vi "RT_Control_Adrian_ESP_NoTrigger.vi"(10 "rt fifo":refnum<k33>, 11 "Parameters":T1={"N_chan"=0, "Input Rate (Hz)"=0.0, "Acq Time (s)"=0.0, "NumOfWarmupIters"=0, "Size fifo"=0, "Period NCL (ms)"=0, "Timeout fifo Read"=0, "Size Sent Array"=0, "Output offsets"=[], "Input offsets"=[0.0, 0.0, 0.0, 0.0, 0.0, 0.0, 0.0, 0.0]}) -> (0 "error out":errorcluster, 2 "Delayed Cycles":dbl)   [LabVIEW 2021]
uses:
  ClosedLoopFlapV3/parametersRT.ctl
  <vilib>/DAQmx/write.llb/DAQmx Write (Analog 1D DBL NChan 1Samp).vi
  <vilib>/DAQmx/read.llb/DAQmx Read (Analog 1D DBL NChan 1Samp).vi
  <vilib>/DAQmx/configure/timing.llb/DAQmx Timing (Sample Clock).vi
  <vilib>/DAQmx/miscellaneous.llb/DAQmx Fill In Error Info.vi
  <resource>/objmgr/daqmx.rc
panel:
  out "timed out?":bool
  out "# elements":u32
  out "data":dbl[](array[numeric]) format="%0.2f"
  out "Numeric":i32
  out "output array":dbl[](array[numeric])
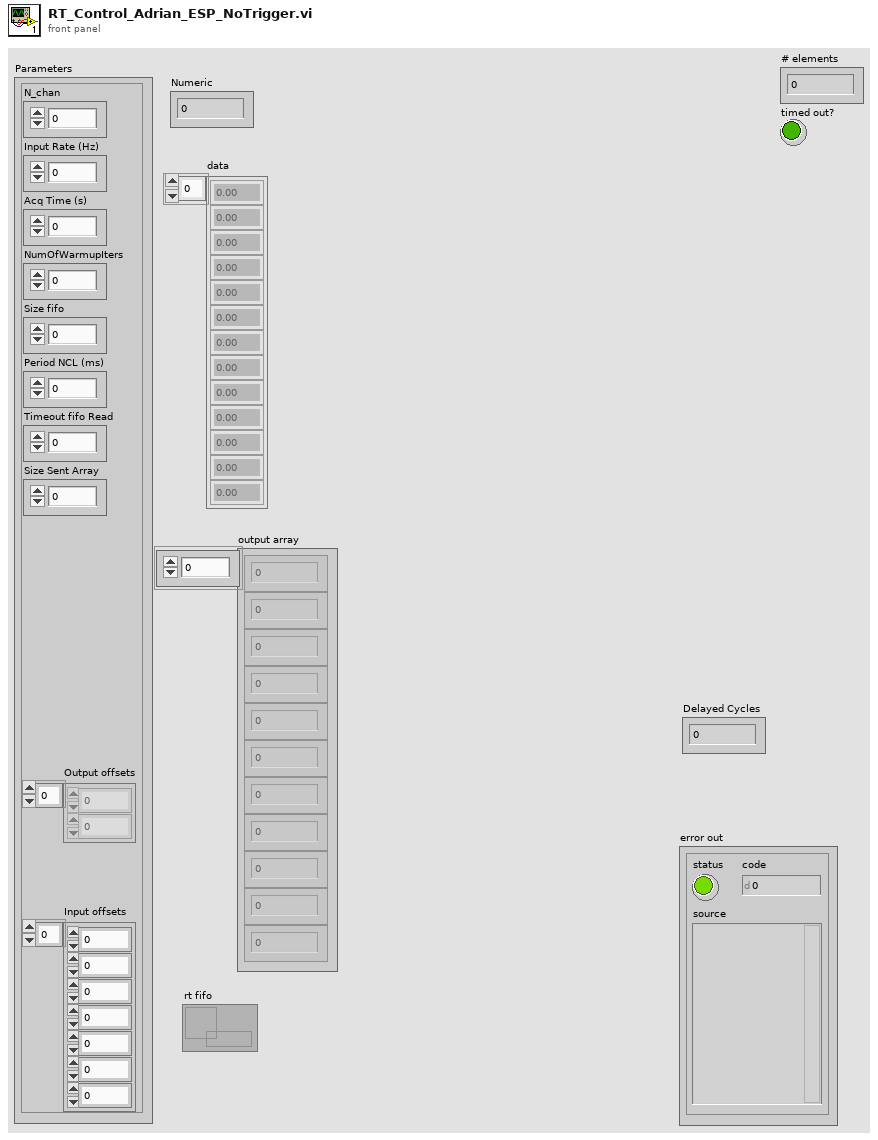
[diagram p1: front panel]
types:
  T1 = typedef "parametersRT.ctl" = cluster{"N_chan":u32, "Input Rate (Hz)":dbl, "Acq Time (s)":dbl, "NumOfWarmupIters":u32, "Size fifo":u32, "Period NCL (ms)":i64, "Timeout fifo Read":i32, "Size Sent Array":i32, "Output offsets":dbl[], "Input offsets":dbl[]}
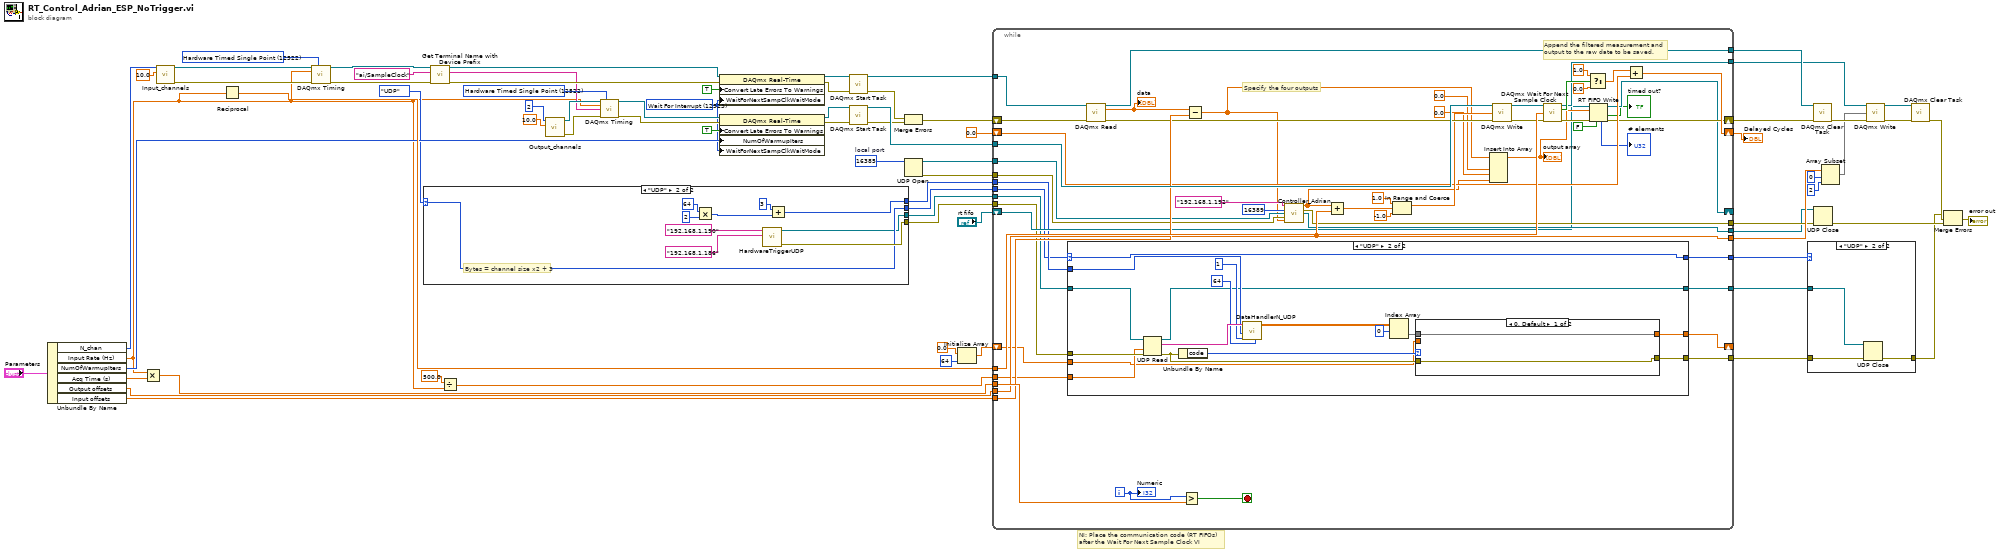
[diagram p0: block diagram]
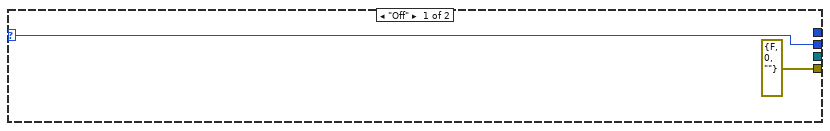
[diagram p3: hidden frame]
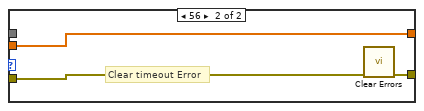
[diagram p5: hidden frame]
diagram:
  w31 = u16 16385  # local port
  w38 = 12522 items=["Finite Samples"=10178, "Continuous Samples"=10123, "Hardware Timed Single Point"=12522] ("sample mode")
  w46 = 12523 items=["Wait For Interrupt"=12523, "Poll"=12524, "Yield"=12525] ("WaitForNextSampClkWaitMode")
  w72 = 12522 items=["Finite Samples"=10178, "Continuous Samples"=10123, "Hardware Timed Single Point"=12522] ("sample mode")
  # "NI: Place the communication code (RT FIFOs) \nafter the Wait For Next Sample Clock VI"
  n1 = Unbundle By Name("Parameters") -> ("N_chan"=w57:u32, "Input Rate (Hz)"=w6:dbl, "NumOfWarmupIters"=w58:u32, "Acq Time (s)"=w65:dbl, "Output offsets"=w56:dbl[], "Input offsets"=w47:dbl[])
  n2 = Multiply(x=w6, y=w65) -> (x*y=w25:dbl)
  n3 = call "Input_channels.vi"("Range"=10.0, "nchan"=w57) -> ("error out"=w40:errorcluster, "Refnum out"=w39:refnum<k21>)  [unwired: 8 in]
  n4 = Reciprocal(x=w6) -> (1/x=w71:dbl)
  n5 = call-poly <vilib>:"DAQmx Timing.vi"("task/channels in"=w39, "sample mode"=w38, "rate"=w6, "error in"=w40) -> ("task out"=w19:refnum<k21>, "error out"=w21:errorcluster)  [unwired: 10 in]
  n6 = case shown="\"UDP\"" enum16{"Off", "UDP"}."UDP" {
    selector: enum16{"Off", "UDP"}."UDP" -> [w75 w78]
    tunnel: [_ w81] -> w12
    tunnel: [errorcluster {"status"=FALSE, "code"=0, "source"=""} ("error constant") w79] -> w14
    tunnel: [w75 w78] -> w11
    tunnel: [_ w77] -> w13
    frame "Off" {
    }
    frame "UDP" {
      # "Bytes = channel size x2 + 3"
      n7 = Multiply(x=64, y=2) -> (x*y=w84:i32)
      n8 = call "HardwareTriggerUDP.vi"("Local IP address"="192.168.1.186" ("Hardware Trigger"), "Remote IP address"="192.168.1.190" ("IP address")) -> ("error out"=w79:errorcluster, "connection ID out"=w77:refnum<k16>)  [unwired: 8 in]
      n9 = Add(x=3, y=w84) -> (x+y=w81:i32)
    }
  }
  n10 = call "Get Terminal Name with Device Prefix.vi"("error in (no error)"=w21, "Local Terminal Name"="ai/SampleClock", "task/channels in"=w19) -> ("error out"=w20:errorcluster, "Terminal Name with Device Prefix"=w17:tag, "task out"=w18:refnum<k21>)  [unwired: 6 in]
  n11 = Divide(x=500.0, y=w6) -> (x/y=w5:dbl)
  n12 = call "Output_channels.vi"("Range"=10.0 ("Maximum Value"), "nchan"=2) -> ("error out"=w62:errorcluster, "Refnum out"=w61:refnum<k21>)  [unwired: 8 in]
  n13 = call-poly <vilib>:"DAQmx Timing.vi"("task/channels in"=w61, "sample mode"=w72, "rate"=w6, "source"=w17, "error in"=w62) -> ("task out"=w70:refnum<k21>, "error out"=w69:errorcluster)  [unwired: 9 in]
  n14 = property class="DAQmx Real-Time"(reference=w18, error in=w20, "Convert Late Errors To Warnings"=TRUE, "WaitForNextSampClkWaitMode"=w46) -> (reference out=w35:refnum<k21>, error out=w34:errorcluster)
  n15 = property class="DAQmx Real-Time"(reference=w70, error in=w69, "Convert Late Errors To Warnings"=TRUE, "NumOfWarmupIters"=w58, "WaitForNextSampClkWaitMode"=w46) -> (reference out=w66:refnum<k21>, error out=w43:errorcluster)
  n16 = call <vilib>:"DAQmx Start Task.vi"("task/channels in"=w35, "error in"=w34) -> ("task out"=w64:refnum<k21>, "error out"=w33:errorcluster)  [unwired: 12 in]
  n17 = call <vilib>:"DAQmx Start Task.vi"("task/channels in"=w66, "error in"=w43) -> ("task out"=w63:refnum<k21>, "error out"=w42:errorcluster)  [unwired: 12 in]
  n18 = Merge Errors(w33, w42) -> (w32:errorcluster)
  n19 = UDP Open(11:w31) -> (port=w29:refnum<k16>, 0:w30:errorcluster)  [unwired: 4 in, 1 out]
  n20 = Initialize Array(0.0, 64) -> (w8:dbl[])
  n21 = while {
    shift-right: [w105] -> w41
    shift-left: w32 -> [w123]
    shift-right: [w135] -> w73
    shift-left: 0.0 ("f") -> [w110]
    tunnel: w71 -> [w133]
    tunnel: w25 -> [w131]
    tunnel: w63 -> [w129]
    tunnel: [w124] -> w67
    tunnel: w64 -> [w125]
    tunnel: [w127] -> w55
    tunnel: w56 -> [w118]
    tunnel: [w118] -> w50
    tunnel: w47 -> [w126]
    tunnel: w30 -> [w116]
    tunnel: w29 -> [w115]
    tunnel: [w114] -> w28
    tunnel: [w113] -> w27
    shift-right: [w101] -> _
    shift-left: "rt fifo" -> [w102]
    tunnel: w14 -> [w95]
    tunnel: w13 -> [w94]
    tunnel: w12 -> [w93]
    tunnel: w11 -> [w92]
    tunnel: w5 -> [w90]
    tunnel: [w89] -> w4
    tunnel: [w88] -> w3
    tunnel: [w87] -> w2
    shift-right: [w86] -> _
    shift-left: w8 -> [w91]
    i -> [w108]
    stop <- w132 stop-if-true
    # "Append the filtered measurement and \noutput to the raw date to be saved."
    # "Specify the four outputs"
    n22 = case shown="\"UDP\"" w92 {
      selector: w92 -> [w142 w156]
      tunnel: w93 -> [_ w158]
      tunnel: w95 -> [w141 w157]
      tunnel: [w141 w150] -> w88
      tunnel: [w142 w156] -> w87
      tunnel: [w139 w146] -> w86
      tunnel: w90 -> [_ w147]
      tunnel: w94 -> [w140 w149]
      tunnel: [w140 w148] -> w89
      tunnel: w91 -> [w139 w145]
      frame "Off", Default {
      }
      frame "UDP" {
        n23 = UDP Read(connection ID=w149, timeout ms (25000)=w147, 8:w157) -> (data out=w159:string, error out=w151:errorcluster, 3:w148:refnum<k16>)  [unwired: 1 in, 2 out]
        n24 = Unbundle By Name(w151) -> ("code"=w152:i32)
        n25 = call "DataHandlerN_UDP.vi"("Data Cycles Per Buffer"=1, "Rx Packet Byte size"=w158, "data out"=w159, "Nchan"=64) -> ("Data"=w143:sgl[][])  [unwired: 1 in, 4 out]
        n26 = Index Array(array=w143, index (row)=0 ("Data Cycles Per Buffer")) -> (element=w144:sgl[])  [unwired: 1 in]
        n27 = case shown="0, Default" w152 {
          tunnel: w151 -> [w161 w164]
          tunnel: [w161 w163] -> w150
          tunnel: w144 -> [w160 _]
          tunnel: [w160 w162] -> w146
          tunnel: w145 -> [_ w162]
          frame 0, Default {
          }
          frame 56 {
            # "Clear timeout Error"
            n28 = call <vilib>:"Clear Errors.vi"("error in (no error)"=w164) -> ("error out"=w163:errorcluster)  [unwired: 5 in, 1 out]
          }
        }
      }
    }
    n29 = call-poly <vilib>:"DAQmx Read.vi"("task/channels in"=w125, "error in"=w123) -> ("task out"=w124:refnum<k21>, "data"=w107:dbl[], "error out"=w122:errorcluster)  [unwired: 11 in]
    "data" <- w107
    n30 = Greater?(x=w108, y=w131) -> (0:w132:bool)
    n31 = Subtract(x=w107, y=w126) -> (x-y=w109:dbl[])
    n32 = call "Controller_Adrian.vi"("name 2"="192.168.1.192", "port or service name"=u16 16389, "connection ID"=w115, "error in (no error)"=w116, "x"=w109) -> ("*(type *) &x"=w100:dbl[], "error out"=w114:errorcluster, "connection ID out"=w113:refnum<k16>)  [unwired: 8 in]
    n33 = Add(x=w100, y=w118) -> (x+y=w120:dbl[])
    n34 = In Range and Coerce(upper limit=1.0, x=w120, lower limit=-1.0) -> (coerced(x)=w117:dbl[])  [unwired: 1 out]
    n35 = Insert Into Array(array=w109, new element #1=0.0 ("new element/subarray"), new element #2=0.0 ("new element/subarray"), new element #3=w100) -> (w103:dbl[])  [unwired: 1 in]
    "output array" <- w103
    n36 = call-poly <vilib>:"DAQmx Write.vi"("task/channels in"=w129, "data"=w117, "error in"=w122) -> ("task out"=w128:refnum<k21>, "error out"=w130:errorcluster)  [unwired: 10 in, 1 out]
    n37 = call <vilib>:"DAQmx Wait For Next Sample Clock.vi"("task/channels in"=w128, "timeout (sec)"=w133, "error in"=w130) -> ("task out"=w127:refnum<k21>, "is late?"=w134:bool, "error out"=w104:errorcluster)  [unwired: 10 in]
    n38 = Select(t=1.0, s=w134, f=0.0) -> (s? t:f=w136:dbl)
    n39 = RT FIFO Write(0:w102, 1:w103, 3:w104, 5:FALSE ("overwrite on timeout (T)")) -> (7:→"# elements":u32, 8:w101:refnum<k33>, 10:→"timed out?":bool, 11:w105:errorcluster)  [unwired: 1 in]
    n40 = Add(x=w136, y=w110) -> (x+y=w135:dbl)
    "Numeric" <- w108
  }
  "Delayed Cycles" <- w73
  n41 = case shown="\"UDP\"" w2 {
    tunnel: w3 -> [w165 w168]
    tunnel: [w165 w167] -> w1
    tunnel: w4 -> [_ w166]
    frame "Off", Default {
    }
    frame "UDP" {
      n42 = UDP Close(connection ID=w166, 8:w168) -> (error out=w167:errorcluster)  [unwired: 1 out]
    }
  }
  n43 = call <vilib>:"DAQmx Clear Task.vi"("task in"=w67, "error in"=w41) -> ("error out"=w53:errorcluster)  [unwired: 13 in]
  n44 = UDP Close(connection ID=w27, 8:w28) -> (error out=w26:errorcluster)  [unwired: 1 out]
  n45 = Array Subset(array=w50, index=0, length=2) -> (w51:dbl[])
  n46 = call-poly <vilib>:"DAQmx Write.vi"("task/channels in"=w55, "data"=w51, "error in"=w53) -> ("task out"=w54:refnum<k21>, "error out"=w52:errorcluster)  [unwired: 10 in, 1 out]
  n47 = call <vilib>:"DAQmx Clear Task.vi"("task in"=w54, "error in"=w52) -> ("error out"=w45:errorcluster)  [unwired: 13 in]
  n48 = Merge Errors(w1, w45, w26) -> (→"error out":errorcluster)
